vi "Div Scalar.vi"(1 "Digits":i32, 2 "Scalar":i32, 3 "A":T1={"Array Num"=[1, 2, 3], "Decimal Index"=0, "stop"=FALSE}) -> (0 "A / Scalar":T1={"Array Num"=[1, 2, 3], "Decimal Index"=0, "stop"=FALSE})   [LabVIEW 2025]
uses:
  Number.ctl
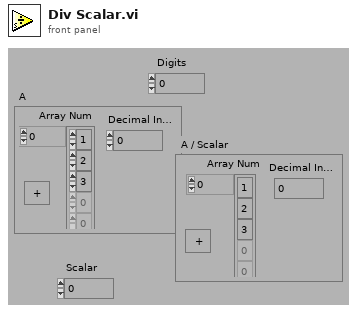
[diagram p1: front panel]
types:
  T1 = typedef "Number.ctl" = cluster{"Array Num":i8[], "Decimal Index":i32, "stop":bool}
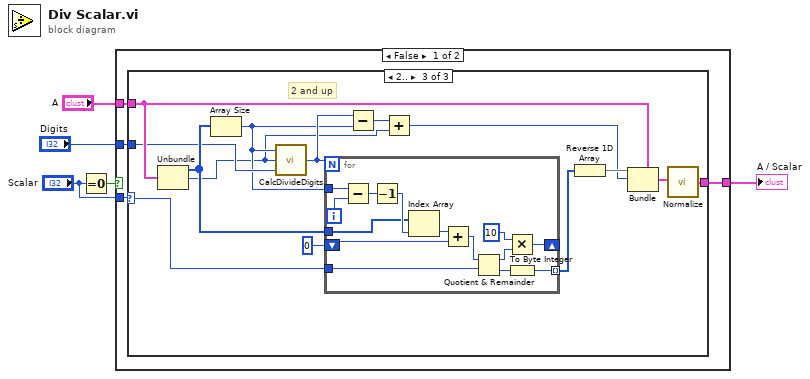
[diagram p0: block diagram]
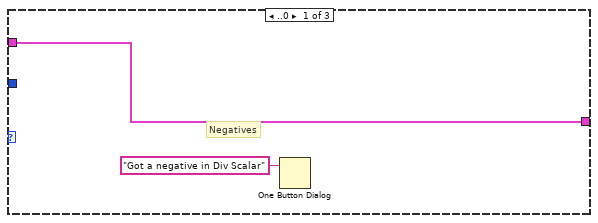
[diagram p2: hidden frame]
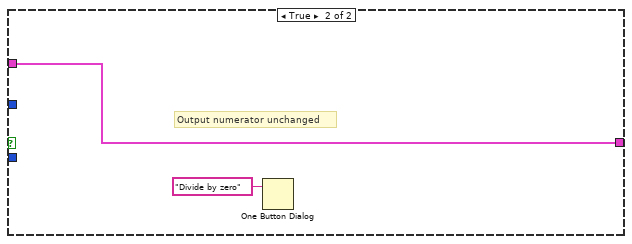
[diagram p4: hidden frame]
diagram:
  n1 = Equal To 0?(x="Scalar") -> (x = 0?=w5:bool)
  n2 = case shown="False" w5 {
    tunnel: "Scalar" -> [w8 _]
    tunnel: "A" -> [w9 w42]
    tunnel: [w7 w42] -> w2
    tunnel: "Digits" -> [w6 _]
    frame False {
      n3 = case shown="2.." w8 {
        selector: w8 -> [_ _ w23]
        tunnel: w9 -> [w11 w12 w21]
        tunnel: [w11 w12 w26] -> w7
        tunnel: w6 -> [_ _ w18]
        frame ..0 {
          # "Negatives"
          n4 = One Button Dialog(message="Got a negative in Div Scalar") -> ()  [unwired: 1 in, 1 out]
        }
        frame 1 {
          # "Just output numerator"
        }
        frame 2.. {
          # "2 and up"
          n5 = Unbundle(w21) -> ("Array Num"=w22:i8[], "Decimal Index"=w14:i32)  [unwired: 1 out]
          n6 = Array Size(array=w22) -> (size(s)=w16:i32)
          n7 = call "CalcDivideDigits.vi"("Digits"=w18, "decimal Ofst"=w14, "Array Size"=w16) -> ("decimal Ofst 2"=w17:i32)
          n8 = for {
            N: w17 -> [_]
            tunnel: w22 -> [w30]
            tunnel: w23 -> [w40]
            tunnel: [w28] -> w20 mode=indexing
            shift-right: [w34] -> _
            shift-left: 0 -> [w38]
            tunnel: w16 -> [w27]
            i -> [w32]
            n9 = Subtract(x=w27, y=w32) -> (x-y=w33:i32)
            n10 = Decrement(x=w33) -> (x-1=w31:i32)
            n11 = Index Array(array=w30, index=w31) -> (element=w29:i8)
            n12 = Add(x=w29, y=w38) -> (x+y=w37:i32)
            n13 = Quotient & Remainder(x=w37, y=w40) -> (x-y*floor(x/y)=w35:i32, floor(x/y)=w39:i32)
            n14 = Multiply(x=10, y=w35) -> (x*y=w34:i32)
            n15 = To Byte Integer(number=w39) -> (8bit integer=w28:i8)
          }
          n16 = Subtract(x=w17, y=w16) -> (x-y=w15:i32)
          n17 = Add(x=w15, y=w14) -> (x+y=w13:i32)
          n18 = Reverse 1D Array(array=w20) -> (reversed array=w19:i8[])
          n19 = Bundle(cluster=w21, "Array Num"=w19, "Decimal Index"=w13) -> (w25:T1)  [unwired: 1 in]
          n20 = call "Normalize.vi"("A"=w25) -> ("Normalized A"=w26:T1)  [unwired: 1 in]
        }
      }
    }
    frame True {
      # "Output numerator unchanged"
      n21 = One Button Dialog(message="Divide by zero") -> ()  [unwired: 1 in, 1 out]
    }
  }
  "A / Scalar" <- w2
